vi "Run VI Transparently.vi"(7 "Run Transparently? (T)":bool=TRUE, 8 "error in":errorcluster, 11 "vi path":path) -> (0 "error out":errorcluster)   [LabVIEW 2011]
uses:
  Controls/TransparencyEffectOperations.ctl
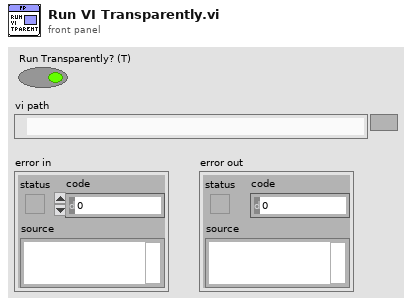
[diagram p1: front panel]
types:
  T1 = typedef "TransparencyEffectOperations.ctl" = enum16{"Show", "Hide 80%", "Hide All"}
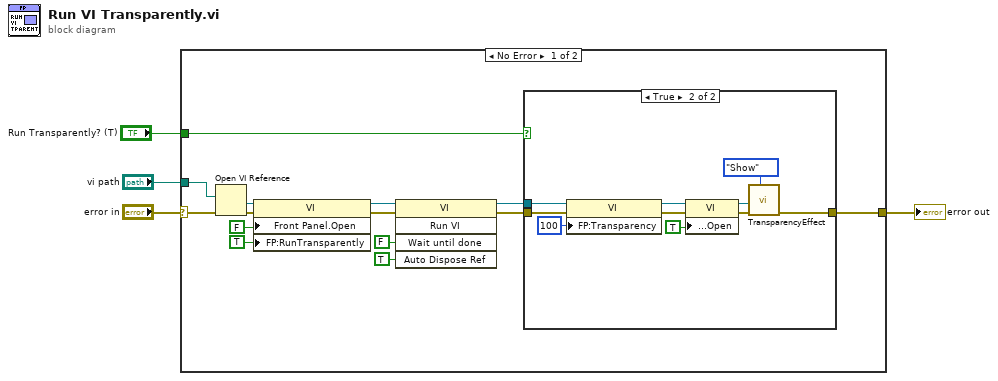
[diagram p0: block diagram]
diagram:
  n1 = case shown="No Error" "error in" {
    selector: "error in" -> [w6 w30]
    tunnel: [w18 w30] -> w4
    tunnel: "vi path" -> [w12 _]
    tunnel: "Run Transparently? (T)" -> [w5 _]
    frame No Error {
      n2 = Open VI Reference(vi path=w12, error in (no error)=w6) -> (vi reference=w7:refnum<vi>, error out=w9:errorcluster)  [unwired: 4 in]
      n3 = property class="VI"(reference=w7, error in=w9, "Front Panel.Open"=FALSE ("Front Panel Window:Open"), "FP:RunTransparently"=TRUE ("Front Panel Window:Open")) -> (reference out=w13:refnum<vi>, error out=w14:errorcluster)
      n4 = invoke class="VI" method="Run VI"(reference=w13, error in=w14, "Wait until done"=FALSE ("Wait Until Done"), "Auto Dispose Ref"=TRUE ("Auto Dispose Reference")) -> (reference out=w15:refnum<vi>, error out=w17:errorcluster)  [unwired: 1 in, 3 out]
      n5 = case shown="True" w5 {
        tunnel: [w19 w29] -> w18
        tunnel: w17 -> [w19 w28]
        tunnel: w15 -> [_ w27]
        frame False {
        }
        frame True {
          n6 = property class="VI"(reference=w27, error in=w28, "FP:Transparency"=u8 100 ("Front Panel Window:Transparency")) -> (reference out=w23:refnum<vi>, error out=w22:errorcluster)
          n7 = property class="VI"(reference=w23, error in=w22, "Front Panel.Open"=TRUE ("Wait Until Done")) -> (reference out=w24:refnum<vi>, error out=w26:errorcluster)
          n8 = call "TransparencyEffect.vi"("Operation"=TransparencyEffectOperations."Show", "error in"=w26, "VI Ref in"=w24) -> ("error out"=w29:errorcluster)  [unwired: 8 in]
        }
      }
    }
    frame Error {
    }
  }
  "error out" <- w4
